vi "Pose2D_send.vi"(6 "连接ID":refnum<k5>, 8 "msg.theta":dbl, 9 "msg.y":dbl, 10 "msg.x":dbl, 11 "topic":string="/chatter") -> (0 "连接ID输出":refnum<k5>)   [LabVIEW 2014]
panel:
  out "JSON":string
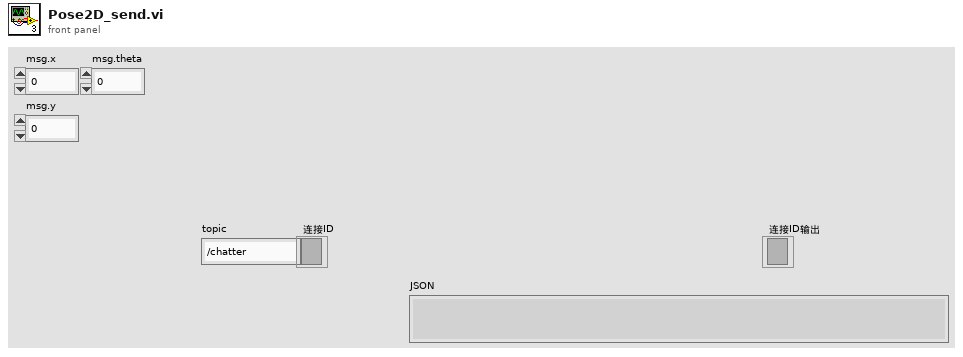
[diagram p1: front panel]
types:
  T1 = cluster{"op":string, "topic":string, "msg":cluster{"x":dbl, "y":dbl, "theta":dbl}}
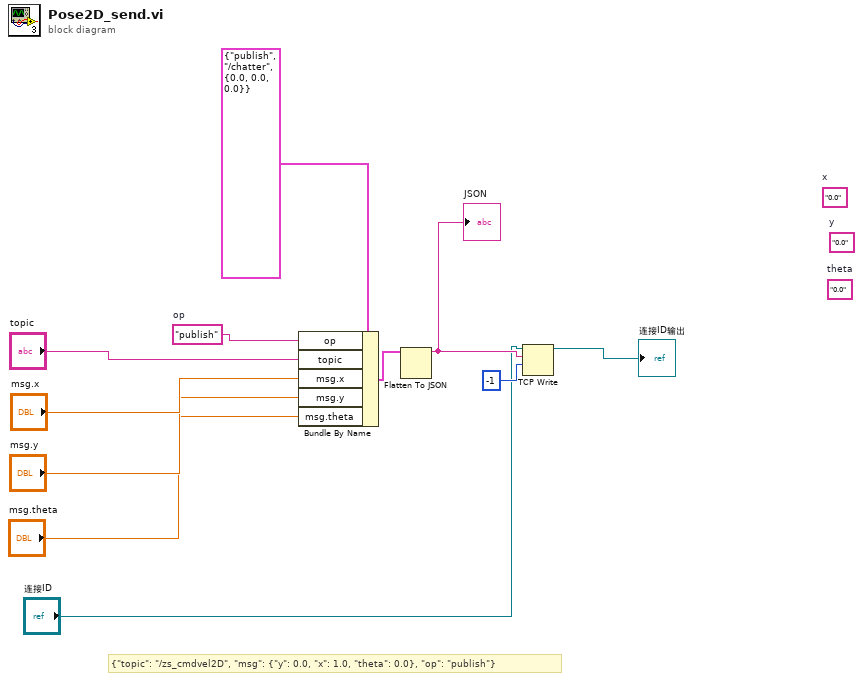
[diagram p0: block diagram]
diagram:
  (unwired) "0.0"  # theta
  (unwired) "0.0"  # y
  (unwired) "0.0"  # x
  w10 = "publish"  # op
  # "{\"topic\": \"/zs_cmdvel2D\", \"msg\": {\"y\": 0.0, \"x\": 1.0, \"theta\": 0.0}, \"op\": \"publish\"}"
  n1 = Bundle By Name(cluster=T1 {"op"="publish", "topic"="/chatter", "msg"={"x"=0.0, "y"=0.0, "theta"=0.0}}, "op"=w10, "topic"="topic", "msg.x"="msg.x", "msg.y"="msg.y", "msg.theta"="msg.theta") -> (w7:T1)
  n2 = Flatten To JSON(anything=w7) -> (JSON string=w5:string)  [unwired: 2 in, 1 out]
  "JSON" <- w5
  n3 = TCP Write(connection ID="连接ID", data in=w5, 9:-1 ("超时毫秒(25000)")) -> (connection ID out=→"连接ID输出":refnum<k5>)  [unwired: 1 in, 2 out]
